vi "Pre-loop init.vi"(8 "error in (no error)":errorcluster, 11 "VI in":refnum<vi>) -> (0 "error out":errorcluster)   [LabVIEW 2018]
doc: "Sets up the messaging and stop event for module."
uses:
  Template Module.lvlib
  ctl/Queue action--enum.ctl
  Modules/Common/Action--enum.ctl
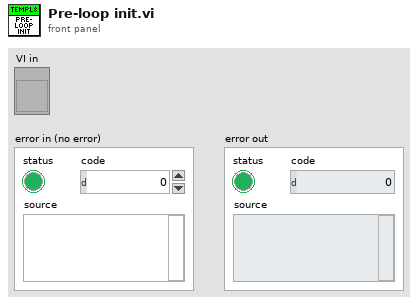
[diagram p1: front panel]
types:
  T1 = typedef "Common.lvlib/Action--enum.ctl" = enum16{"Destroy", "Get", "Stop All Modules", "Create"}
  T2 = typedef "Template Module.lvlib/Queue action--enum.ctl" = enum16{"Create", "Get", "Destroy"}
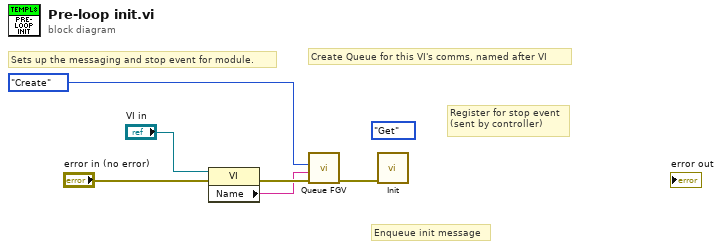
[diagram p0: block diagram]
diagram:
  (unwired) Action--enum."Get" ("Action")
  # "Sets up the messaging and stop event for module."
  # "Enqueue init message"
  # "Register for stop event\n(sent by controller)"
  # "Create Queue for this VI's comms, named after VI"
  n1 = property class="VI"(reference="VI in", error in="error in (no error)") -> (error out=w4:errorcluster, "Name"=w2:string)  [unwired: 1 out]
  n2 = call "Queue FGV.vi"("error in"=w4, "Queue name (unnamed)"=w2, "Queue Action"=Queue_action--enum."Create") -> ("error out"=w6:errorcluster)  [unwired: 7 in, 1 out]
  n3 = call "Init.vi"("error in (no error)"=w6) -> ()  [unwired: 10 in, 1 out]
